vi "DtCreateCtrContMeasureChan.vi"(1 "Start Edge":i32(ring)=752 items=["GateRising"=750, "GateFalling"=751, "ClockRising"=752, "ClockFalling"=753, "AdcConversionComplete"=754, "TachInputFalling"=755, "TachInputRising"=756, "DigitalIn0Falling"=757, "DigitalIn0Rising"=758, "DigitalIn1Falling"=759, "DigitalIn1Rising"=760, "DigitalIn2Falling"=761, "DigitalIn2Rising"=762, "DigitalIn3Falling"=763, "DigitalIn3Rising"=764, "DigitalIn4Falling"=765, "DigitalIn4Rising"=766, "DigitalIn5Falling"=767, "DigitalIn5Rising"=768, "DigitalIn6Falling"=769, "DigitalIn6Rising"=770, "DigitalIn7Falling"=771, "DigitalIn7Rising"=772, "Ct0ClockFalling"=773, "Ct0ClockRising"=774, "Ct0GateFalling"=775, "Ct0GateRising"=776], 2 "Stop Edge":i32(ring)=752 items=["GateRising"=750, "GateFalling"=751, "ClockRising"=752, "ClockFalling"=753, "AdcConversionComplete"=754, "TachInputFalling"=755, "TachInputRising"=756, "DigitalIn0Falling"=757, "DigitalIn0Rising"=758, "DigitalIn1Falling"=759, "DigitalIn1Rising"=760, "DigitalIn2Falling"=761, "DigitalIn2Rising"=762, "DigitalIn3Falling"=763, "DigitalIn3Rising"=764, "DigitalIn4Falling"=765, "DigitalIn4Rising"=766, "DigitalIn5Falling"=767, "DigitalIn5Rising"=768, "DigitalIn6Falling"=769, "DigitalIn6Rising"=770, "DigitalIn7Falling"=771, "DigitalIn7Rising"=772, "Ct0ClockFalling"=773, "Ct0ClockRising"=774, "Ct0GateFalling"=775, "Ct0GateRising"=776], 5 "Board Name":string, 7 "Counter Num":u32, 11 "error in (no error)":errorcluster) -> (4 "Task out":i32, 15 "error out":errorcluster)   [LabVIEW 2016]
doc: "Creates one or more virtual counter/timer channels that measure the time, in milliseconds, between a specified start edge and stop edge of the counter's clock or gate input signal; then, unlike the DtOLCreateTask - Time Between Edges VI, automatically restarts the next measurement.\n\nThe start edge and the stop edge can occur on the rising edge of the gate input signal, the falling edge of the gate input signal, the rising edge of the clock input signal, or the falling edge of the clock input signal.\n\nThis type of task is also called continuous edge-to-edge measurement. To use this VI, your device must support continuous edge-to-edge measurement mode.\n\nOnce you have created a virtual counter/timer channel for a continuous edge-to-edge measurement task, you can start the task and read the measurement using the DtOLRead (Read Single Channel - Single Sample) VI. Note that if you read the counter/timer before the measurement is complete, 0 is returned.\n\nIf your device allows you to stream counter/timer data through an analog input subsystem, you can use this VI to configure the counter/timer channel before you add it to the analog input task."
uses:
  <userlib>/LV-Link3/DtLvLink.lvlib
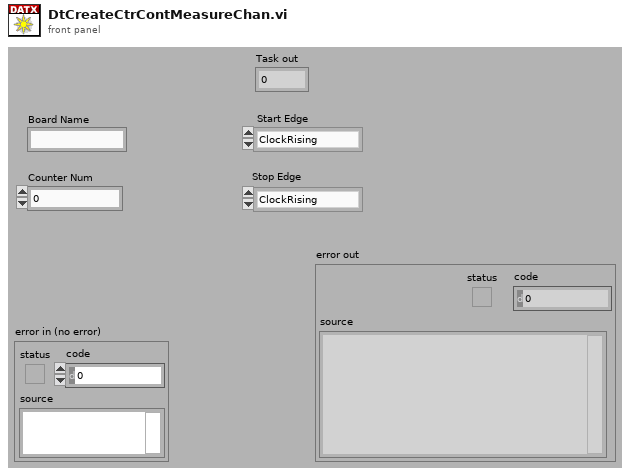
[diagram p1: front panel]
types:
  T1 = enum32{"AnalogInput", "AnalogOutput", "DigitalInput", "DigitalOutput", "Quadrature", "CounterTimer"}
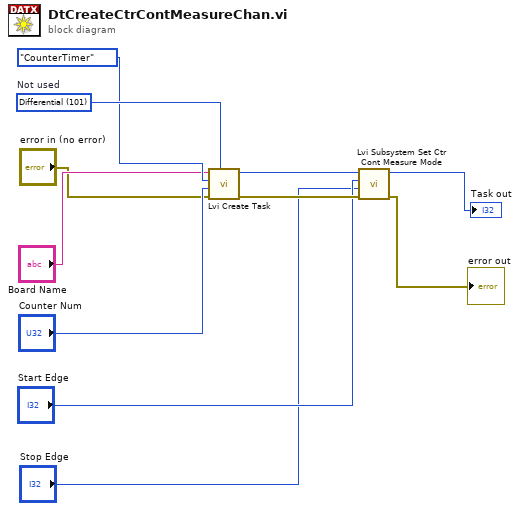
[diagram p0: block diagram]
diagram:
  w6 = 101 items=["SingleEnded"=100, "Differential"=101]  # Not used
  n1 = call <userlib>:"Lvi Create Task.vi"("SEorDiff"=w6, "error in (no error)"="error in (no error)", "SubSysIndex"="Counter Num", "ChanType"=T1."CounterTimer", "BoardName"="Board Name") -> ("error out"=w11:errorcluster, "TaskRef"=w1:i32)  [unwired: 4 in, 1 out]
  n2 = call <userlib>:"Lvi Subsystem Set Ctr Cont Measure Mode.vi"("error in (no error)"=w11, "StopEdge"="Stop Edge", "StartEdge"="Start Edge", "TaskRef"=w1) -> ("error out"=→"error out":errorcluster, "TaskRef out"=→"Task out":i32)  [unwired: 5 in, 1 out]
